vi "Update Values.vi"(6 "Timestamp (Now)":dbl, 8 "error in (no error)":errorcluster, 9 "Raw Values (N/A)":dbl[](array[numeric]), 10 "Values":dbl[](array[numeric]), 11 "Group in":refnum<class "Group.lvclass">) -> (0 "error out":errorcluster, 3 "Group out":refnum<class "Group.lvclass">)   [LabVIEW 2020, in "Vecto.lvlib" / "Group.lvclass"]
uses:
  Group.lvclass
  C:/dev/lv20CE/relink/lv-vecto/Vecto/GroupAbstract/GroupAbstract.lvclass
  Group.lvclass/Group.ctl
  GroupAbstract/GroupAbstract.lvclass
  C:/dev/lv20CE/relink/lv-vecto/Vecto/Group/Group.lvclass
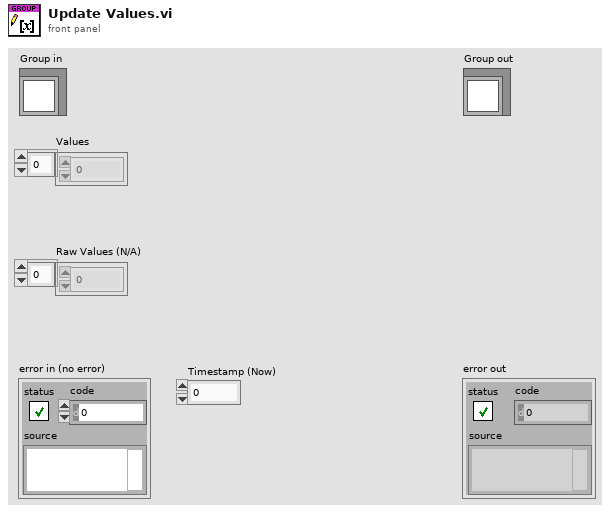
[diagram p1: front panel]
types:
  T1 = typedef "Vecto.lvlib/Group.lvclass/Ref.ctl" = cluster{"Scaled":dbl[], "Timestamp":dbl[], "Raw":dbl[]}
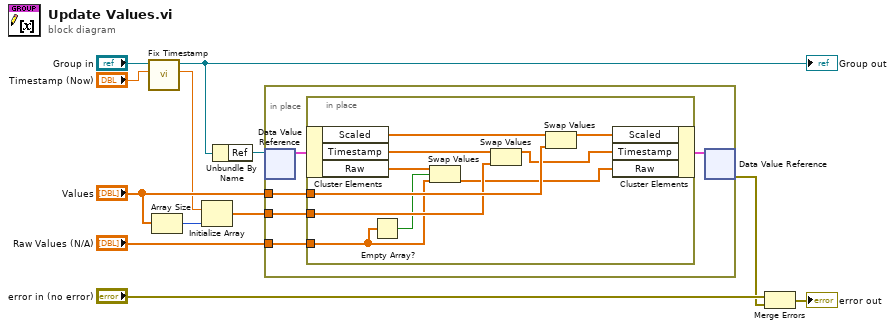
[diagram p0: block diagram]
diagram:
  n1 = call "Fix Timestamp.vi"("Timestamp in"="Timestamp (Now)", "GroupAbstract in"="Group in") -> ("Timestamp"=w1:dbl, "GroupAbstract out"=w3:refnum<class "Group.lvclass">)  [unwired: 7 in, 1 out]
  "Group out" <- w3
  n2 = Array Size(array="Values") -> (size(s)=w5:i32)
  n3 = Initialize Array(w1, w5) -> (w4:dbl[])
  n4 = Unbundle By Name(w3) -> ("Ref"=w10:refnum<data-value>)
  n5 = in-place {
    in-place-border: "Values" -> [w17]
    in-place-border: "Raw Values (N/A)" -> [w15]
    in-place-border: w4 -> [w16]
    n6 = in-place-dvr #1(w10) -> (w14:T1)  [unwired: 1 out]
    n7 = in-place {
      in-place-border: w17 -> [w26]
      in-place-border: w16 -> [w22]
      in-place-border: w15 -> [w19]
      n8 = in-place-cluster #2(w14) -> ("Scaled"=w27:dbl[], "Timestamp"=w24:dbl[], "Raw"=w23:dbl[])
      n9 = Empty Array?(array=w19) -> (empty?=w18:bool)
      n10 = Swap Values(12:w23, 13:w18, 14:w19) -> (3:w20:dbl[])  [unwired: 1 out]
      n11 = Swap Values(12:w24, 14:w22) -> (1:w21:dbl[])  [unwired: 1 in, 1 out]
      n12 = Swap Values(12:w27, 14:w26) -> (1:w25:dbl[])  [unwired: 1 in, 1 out]
      n13 = in-place-cluster #2("Scaled"=w25, "Timestamp"=w21, "Raw"=w20) -> (w13:T1)
    }
    n14 = in-place-dvr #1(w13) -> (w7:errorcluster)  [unwired: 1 out]
  }
  n15 = Merge Errors("error in (no error)", w7) -> (→"error out":errorcluster)
